vi "MotionDetected_glob.vi"() -> ()   [LabVIEW 2021]
panel:
  in  "Motion Detected":u16(ring) items=["reflector spin", "downward slash", "overhead block", "-none-"]
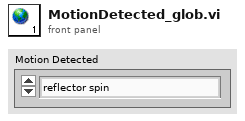
[diagram p1: front panel]
diagram:
